vi "USER_EDITOR_prepare_SELECT_statement.vi"(7 "nmb_of_top_rows (all)":i32, 8 "error_in":errorcluster) -> (0 "error_out":errorcluster, 3 "SELECT_statement":string)   [LabVIEW 2019]
uses:
  FGV/USER_EDITOR_records_display/FGV_USER_EDITOR_records_display.ctl
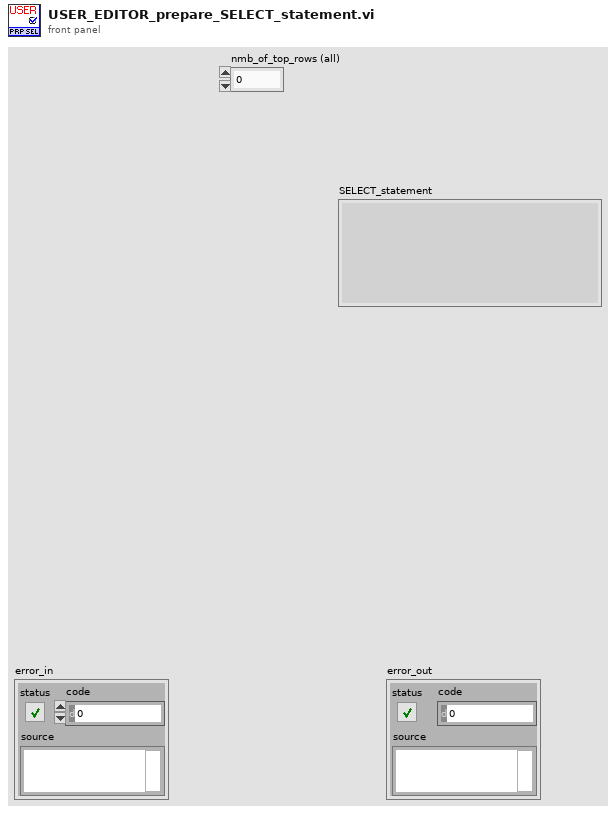
[diagram p1: front panel]
types:
  T1 = typedef "FGV_USER_EDITOR_records_display.ctl" = enum16{"initialize", "set_user_edit_tables_names", "set_headers", "set_records", "get_user_edit_table_name", "get_user_edit_hist_table_name", "get_headers", "get_uneditable_columns", "get_all_info", "record_added?", "record_inserted?", "record_edited?", "record_updated?", "record_deleted?", "discard_changes"}
  T2 = typedef "USER_EDITOR_all_info.ctl" = cluster{"user_table":string, "user_history":string, "headers":string[], "uneditable_columns":string[], "uneditable_columns":i32[], "editable_columns":i32[], "values_in_database":string[][], "size":cluster{"columns":i32, "SQL_rows":i32, "disp_rows":i32}, "USER_record_states":T3[]}
  T3 = typedef "SQL_record_states.ctl" = enum16{"Equal", "Added", "Edited", "Deleted"}
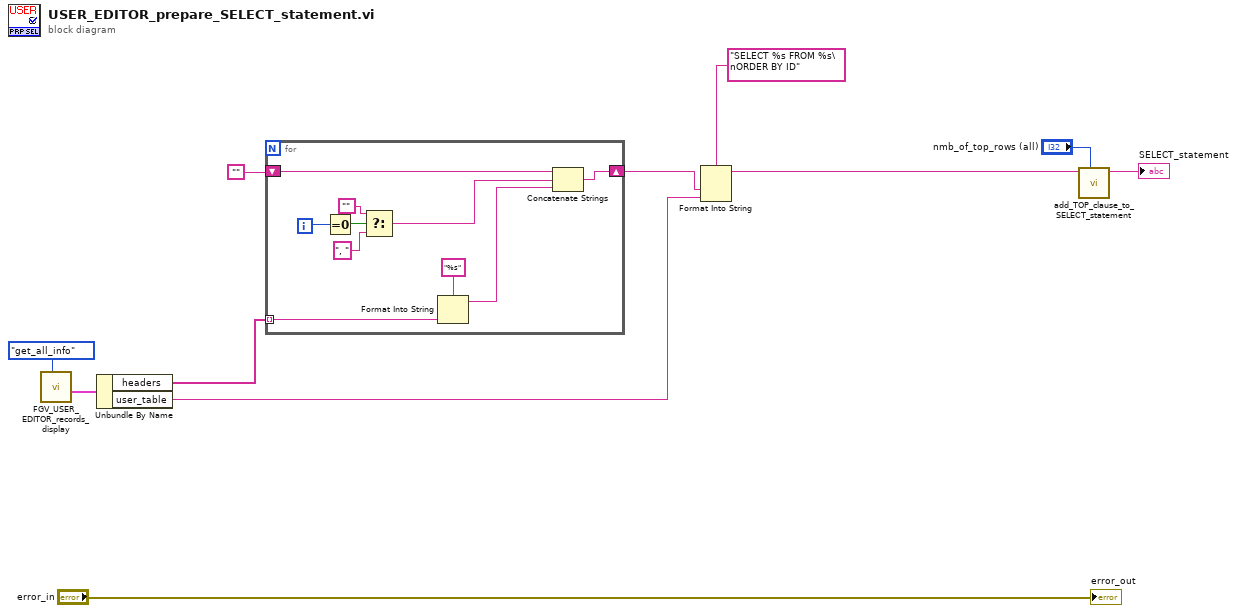
[diagram p0: block diagram]
diagram:
  n1 = call "FGV_USER_EDITOR_records_display.vi"("options"=FGV_USER_EDITOR_records_display."get_all_info") -> ("all_info"=w1:T2)  [unwired: 7 in, 3 out]
  n2 = Unbundle By Name(w1) -> ("headers"=w8:string[], "user_table"=w5:string)
  n3 = for {
    tunnel: w8 -> [w14] mode=indexing
    shift-right: [w16] -> w6
    shift-left: "" -> [w17]
    i -> [w21]
    n4 = Equal To 0?(x=w21) -> (x = 0?=w20:bool)
    n5 = Select(t="", s=w20, f=", ") -> (s? t:f=w15:string)
    n6 = Format Into String(format string="%s", w14) -> (resulting string=w13:string)  [unwired: 2 in, 1 out]
    n7 = Concatenate Strings(w17, w15, w13) -> (w16:string)
  }
  n8 = Format Into String(format string="SELECT %s FROM %s\nORDER BY ID", w6, w5) -> (resulting string=w4:string)  [unwired: 2 in, 1 out]
  n9 = call "add_TOP_clause_to_SELECT_statement.vi"("nmb_of_top_rows (all)"="nmb_of_top_rows (all)", "SELECT_statement_in"=w4) -> ("SELECT_statement_out"=→"SELECT_statement":string)  [unwired: 8 in, 1 out]
  "error_out" <- "error_in"
